vi "RSZVB Set Display Line.vi"(7 "Position (0.0)":dbl format="%^.3e", 8 "error in (no error)":errorcluster {"code" format="%.0x"}, 9 "Display Line (F: Off)":bool, 10 "Channel (Trace) (1)":i32=1, 11 "VISA session":refnum<visa-resource-name>) -> (0 "error out":errorcluster {"code" format="%.0x"}, 3 "dup VISA session":refnum<visa-resource-name>)   [LabVIEW 2011]
doc: "This VI shows or hides the display line associated to the active trace in a Cartesian diagram area.\n\nRemote-control command(s):\nCALCulate<Ch/Tr>:DLINe:STATe <Boolean>\nCALCulate<Ch/Tr>:DLINe <numeric_value>"
panel:
  # "On\nOff"
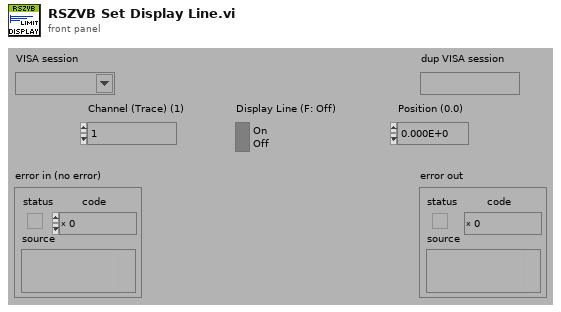
[diagram p1: front panel]
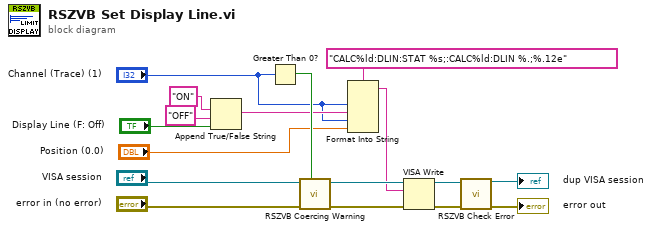
[diagram p0: block diagram]
diagram:
  n1 = Append True/False String(1:"Display Line (F: Off)", 2:"OFF", 3:"ON") -> (0:w3:string)  [unwired: 1 in]
  n2 = Greater Than 0?(x="Channel (Trace) (1)") -> (x > 0?=w4:bool)
  n3 = call "RSZVB Coercing Warning.vi"("In Range?"=w4, "error in (no error)"="error in (no error)", "VISA session"="VISA session") -> ("error out"=w15:errorcluster, "dup VISA session"=w16:refnum<visa-resource-name>)  [unwired: 7 in]
  n4 = Format Into String(format string="CALC%ld:DLIN:STAT %s;:CALC%ld:DLIN %.;%.12e", "Channel (Trace) (1)", w3, "Channel (Trace) (1)", "Position (0.0)") -> (resulting string=w12:string)  [unwired: 2 in, 1 out]
  n5 = VISA Write(VISA resource name=w16, write buffer=w12, error in (no error)=w15) -> (VISA resource name out=w13:refnum<visa-resource-name>, error out=w14:errorcluster)  [unwired: 1 out]
  n6 = call "RSZVB Check Error.vi"("error in (no error)"=w14, "VISA session"=w13) -> ("error out"=→"error out":errorcluster, "dup VISA session"=→"dup VISA session":refnum<visa-resource-name>)  [unwired: 8 in]
